vi "Update UI per Reference.vi"(8 "error in (no error)":errorcluster, 11 "Analyze Results Base in":refnum<class "Analyze Results Base.lvclass">) -> (0 "error out":errorcluster, 3 "Analyze Results Base out":refnum<class "Analyze Results Base.lvclass">)   [LabVIEW 2014, in "Analyze Results Base.lvclass"]
uses:
  Analyze Results Base.lvclass
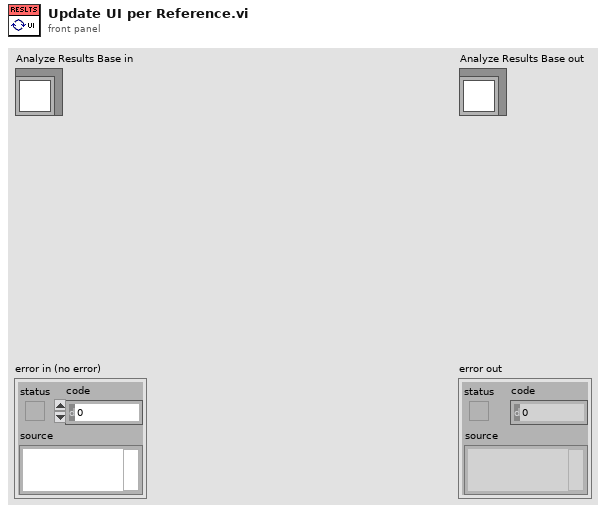
[diagram p1: front panel]
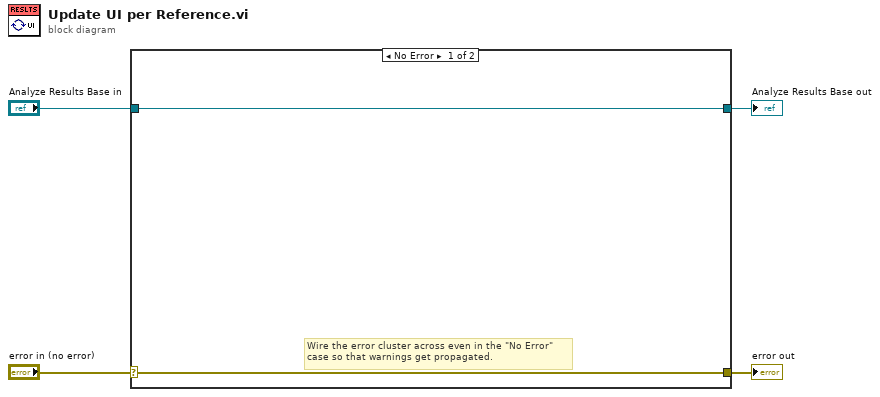
[diagram p0: block diagram]
diagram:
  n1 = case shown="No Error" "error in (no error)" {
    selector: "error in (no error)" -> [w5 w8]
    tunnel: [w5 w8] -> w3
    tunnel: [w6 w7] -> w1
    tunnel: "Analyze Results Base in" -> [w6 w7]
    frame No Error {
      # "Wire the error cluster across even in the \"No Error\"\ncase so that warnings get propagated."
    }
    frame Error {
    }
  }
  "error out" <- w3
  "Analyze Results Base out" <- w1
